vi "Create Calendar.vi"(8 "date time rec":T1, 9 "Month Name":refnum<vi>, 10 "Dates":refnum<vi>, 11 "Display State In":cluster{"Month":i32, "Day":i32, "Year":i32}) -> ()   [LabVIEW 2019, in "Custom Calendar.xctl"]
uses:
  Custom Calendar.xctl
  <vilib>/Utility/miscctls.llb/LVRowAndColumnTypeDef.ctl
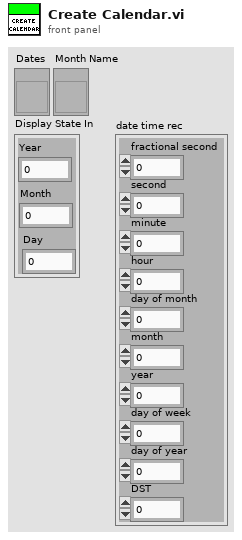
[diagram p1: front panel]
types:
  T1 = cluster{"fractional second":dbl, "second":i32, "minute":i32, "hour":i32, "day of month":i32, "month":i32, "year":i32, "day of week":i32, "day of year":i32, "DST":i32}
  T2 = typedef "LVRowAndColumnTypeDef.ctl" = cluster{"Row":i32, "Column":i32}
  T3 = typedef "LVDateTimeRec.ctl" = cluster{"fractional second":dbl, "second":i32, "minute":i32, "hour":i32, "day of month":i32, "month":i32, "year":i32, "day of week":i32, "day of year":i32, "DST":i32}
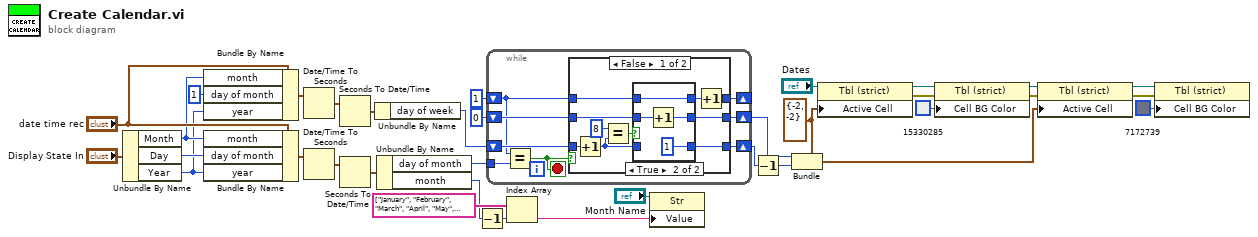
[diagram p0: block diagram]
diagram:
  w6 = T2 {"Row"=-2, "Column"=-2} ("Active Cell:Active Cell")
  n1 = Unbundle By Name("Display State In") -> ("Month"=w18:i32, "Day"=w21:i32, "Year"=w17:i32)
  n2 = Bundle By Name(cluster="date time rec", "month"=w18, "day of month"=1, "year"=w17) -> (w15:T1)
  n3 = Bundle By Name(cluster="date time rec", "month"=w18, "day of month"=w21, "year"=w17) -> (w35:T1)
  n4 = Date/Time To Seconds(2:w15) -> (0:w16:timestamp)  [unwired: 1 in]
  n5 = Date/Time To Seconds(2:w35) -> (0:w34:timestamp)  [unwired: 1 in]
  n6 = Seconds To Date/Time(time stamp (now)=w16) -> (date time rec=w14:T3)  [unwired: 1 in]
  n7 = Seconds To Date/Time(time stamp (now)=w34) -> (date time rec=w33:T3)  [unwired: 1 in]
  n8 = Unbundle By Name(w14) -> ("day of week"=w13:i32)
  n9 = Unbundle By Name(w33) -> ("day of month"=w22:i32, "month"=w28:i32)
  n10 = Decrement(x=w28) -> (x-1=w29:i32)
  n11 = while {
    tunnel: w22 -> [w43]
    shift-right: [w38] -> _
    shift-left: 1 -> [w37]
    shift-right: [w39] -> w25
    shift-left: 0 -> [w40]
    shift-right: [w42] -> w23
    shift-left: w13 -> [w41]
    stop <- w36 stop-if-true
    n12 = Equal?(x=w37, y=w43) -> (x = y?=w36:bool)
    n13 = case shown="False" w36 {
      tunnel: [w52 w61] -> w42
      tunnel: w41 -> [w51 w61]
      tunnel: w40 -> [w50 w62]
      tunnel: [w49 w62] -> w39
      tunnel: [w47 w63] -> w38
      tunnel: w37 -> [w46 w63]
      frame False {
        n14 = Increment(x=w51) -> (x+1=w45:i32)
        n15 = Equal?(x=8 ("y"), y=w45) -> (x = y?=w53:bool)
        n16 = case shown="True" w53 {
          tunnel: [w54 1 ("day of week")] -> w52
          tunnel: w45 -> [w54 _]
          tunnel: w50 -> [w56 w60]
          tunnel: [w56 w59] -> w49
          tunnel: w46 -> [w55 w58]
          tunnel: [w55 w58] -> w48
          frame False {
          }
          frame True {
            n17 = Increment(x=w60) -> (x+1=w59:i32)
          }
        }
        n18 = Increment(x=w48) -> (x+1=w47:i32)
      }
      frame True {
      }
    }
  }
  n19 = Index Array(array=string[] ["January", "February", "March", "April", "May", "June", "July", "August", "September", "October", "November", "December"], index=w29) -> (element=w31:string)
  n20 = property class="Str"(reference="Month Name", "Value"=w31) -> ()  [unwired: 1 in, 2 out]
  n21 = Decrement(x=w23) -> (x-1=w24:i32)
  n22 = Bundle(cluster=w6, "Row"=w25, "Column"=w24) -> (w5:T2)
  n23 = property class="Tbl (strict)"(reference="Dates", "Active Cell"=w6) -> (reference out=w11:refnum<vi>, error out=w9:errorcluster)  [unwired: 1 in]
  n24 = property class="Tbl (strict)"(reference=w11, error in=w9, "Cell BG Color"=u32 15330285 ("Active Cell:Cell Background Color")) -> (reference out=w8:refnum<vi>, error out=w7:errorcluster)
  n25 = property class="Tbl (strict)"(reference=w8, error in=w7, "Active Cell"=w5) -> (reference out=w4:refnum<vi>, error out=w3:errorcluster)
  n26 = property class="Tbl (strict)"(reference=w4, error in=w3, "Cell BG Color"=u32 7172739 ("Active Cell:Cell Background Color")) -> ()  [unwired: 2 out]
